vi "XXPathPlanner_Path_MapPct.vi"(9 "Seg1Pct":dbl, 11 "Pct":dbl) -> (3 "MapPct":dbl)   [LabVIEW 2019]
doc: "Map a given percentage/waypoint relative position over 2 segments This is an internal routine.\n\nInputs: \n - pct - The percent to map\n - seg1Pct - The percentage of the 2 segments made up by the first segment\n\nOutputs:\n - MapPct - The waypoint relative position over the 2 segments"
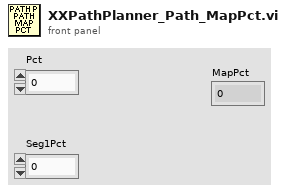
[diagram p1: front panel]
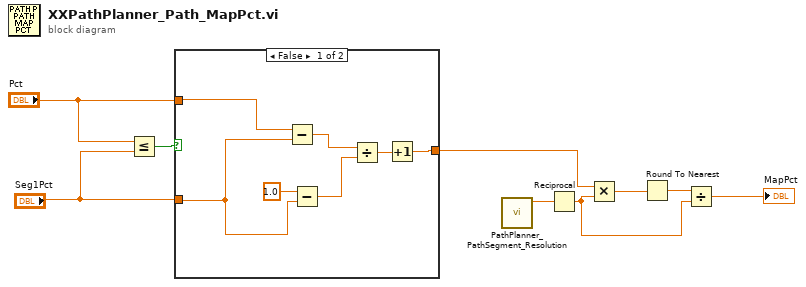
[diagram p0: block diagram]
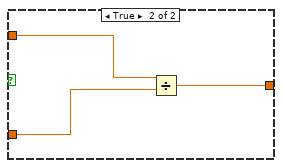
[diagram p2: hidden frame]
diagram:
  n1 = Less Or Equal?(x="Pct", y="Seg1Pct") -> (x <= y?=w9:bool)
  n2 = case shown="False" w9 {
    tunnel: "Pct" -> [w14 w19]
    tunnel: "Seg1Pct" -> [w13 w18]
    tunnel: [w10 w17] -> w5
    frame False {
      n3 = Subtract(x=w14, y=w13) -> (x-y=w12:dbl)
      n4 = Subtract(x=1.0, y=w13) -> (x-y=w15:dbl)
      n5 = Divide(x=w12, y=w15) -> (x/y=w11:dbl)
      n6 = Increment(x=w11) -> (x+1=w10:dbl)
    }
    frame True {
      n7 = Divide(x=w19, y=w18) -> (x/y=w17:dbl)
    }
  }
  n8 = call "PathPlanner_PathSegment_Resolution.vi"() -> ("Resolution"=w6:dbl)  [unwired: 11 in]
  n9 = Reciprocal(x=w6) -> (1/x=w2:dbl)
  n10 = Multiply(x=w5, y=w2) -> (x*y=w4:dbl)
  n11 = Round To Nearest(number=w4) -> (nearest integer value=w3:dbl)
  n12 = Divide(x=w3, y=w2) -> (x/y=→"MapPct":dbl)
